vi "FTW-Test-JobScheduler.vi"() -> (0 "Test Result":errorcluster)   [LabVIEW 2014]
uses:
  src/core/error/FTW-ERR-ThrowError.vi
  src/core/error/FTW-ERR-CallChain.vi
  src/core/string/FTW-STR-ReplaceWhitespace.vi
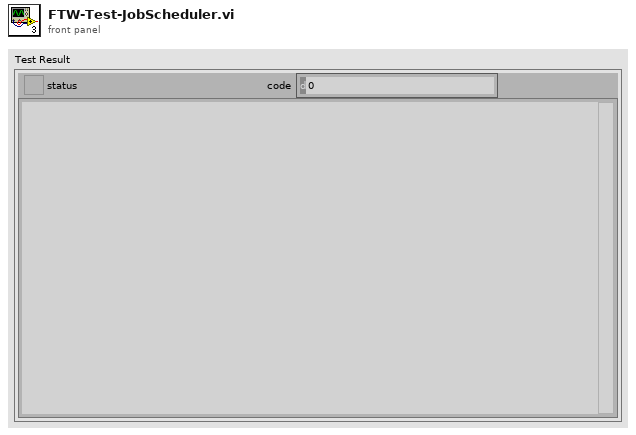
[diagram p1: front panel]
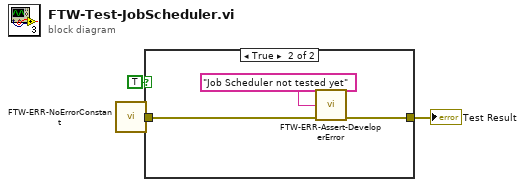
[diagram p0: block diagram]
diagram:
  n1 = call "FTW-ERR-NoErrorConstant.vi"() -> ("no error"=w2:errorcluster)
  n2 = case shown="True" TRUE {
    tunnel: [w4 w6] -> w3
    tunnel: w2 -> [w4 w7]
    frame False {
    }
    frame True {
      n3 = call "FTW-ERR-Assert-DeveloperError.vi"("Reason this error should never happen"="Job Scheduler not tested yet", "error in"=w7) -> ("error out"=w6:errorcluster)  [unwired: 13 in]
    }
  }
  "Test Result" <- w3
